vi "JiLTestR.vi"() -> ()   [LabVIEW 2010]
uses:
  Global 1.vi
panel:
  out "time":dbl
  in  "doublein":dbl(slide) scale=-100.0..100.0
  out "doubleout":dbl
  in  "stringin":string="hola"
  in  "booleanin":bool
  out "booleanout":bool
  out "stringout":string="hola"
  in  "stop":bool
  out "intout":i32
  in  "intin":i32
  # "ESTE ES UN CONTROL REENTRANTE DE LA PLANTA REAL"
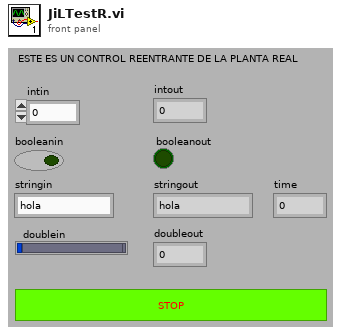
[diagram p1: front panel]
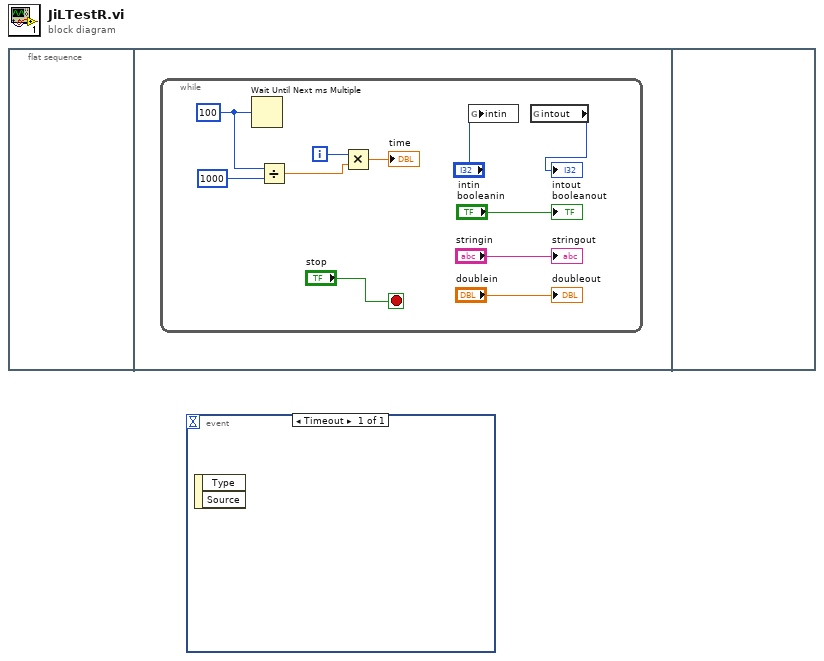
[diagram p0: block diagram]
diagram:
  n1 = flat-sequence {
    frame #0 {
    }
    frame #1 {
      n2 = while {
        i -> [w6]
        stop <- "stop" stop-if-true
        w7 = u32 100 ("millisecond multiple")
        n3 = Wait Until Next ms Multiple(millisecond multiple=w7) -> ()  [unwired: 1 out]
        n4 = Divide(x=w7, y=i64 1000) -> (x/y=w9:dbl)
        n5 = Multiply(x=w6, y=w9) -> (x*y=→"time":dbl)
        n6 = global write "Global 1.vi" "intin"("intin") -> ()
        n7 = global read "Global 1.vi" "intout"() -> (→"intout":i32)
        "stringout" <- "stringin"
        "booleanout" <- "booleanin"
        "doubleout" <- "doublein"
      }
    }
    frame #2 {
    }
  }
  n8 = event shown="[0] Timeout" {
    selector: _ -> [_]
    dyn-events: _ -> [_]
    timeout: _ -> [_]
    event Timeout {
      n9 = event-data() -> ()  [unwired: 1 in, 2 out]
    }
  }
